vi "CrossedLine.vi"(0 "Xpoint1":dbl, 1 "Ypoint1":dbl, 4 "Xpoint2":dbl, 5 "Ypoint2":dbl, 6 "XpointC":dbl, 7 "YpointC":dbl, 8 "XpointP":dbl=-1.0, 9 "YpointP":dbl=-1.0) -> (12 "NextPriorX":dbl, 13 "NextPriorY":dbl, 17 "CrossedLine":bool)   [LabVIEW 2012]
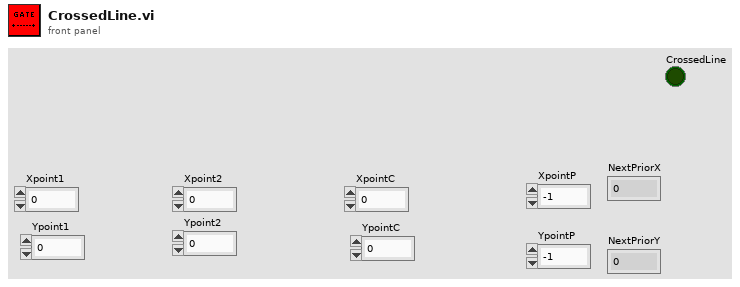
[diagram p1: front panel]
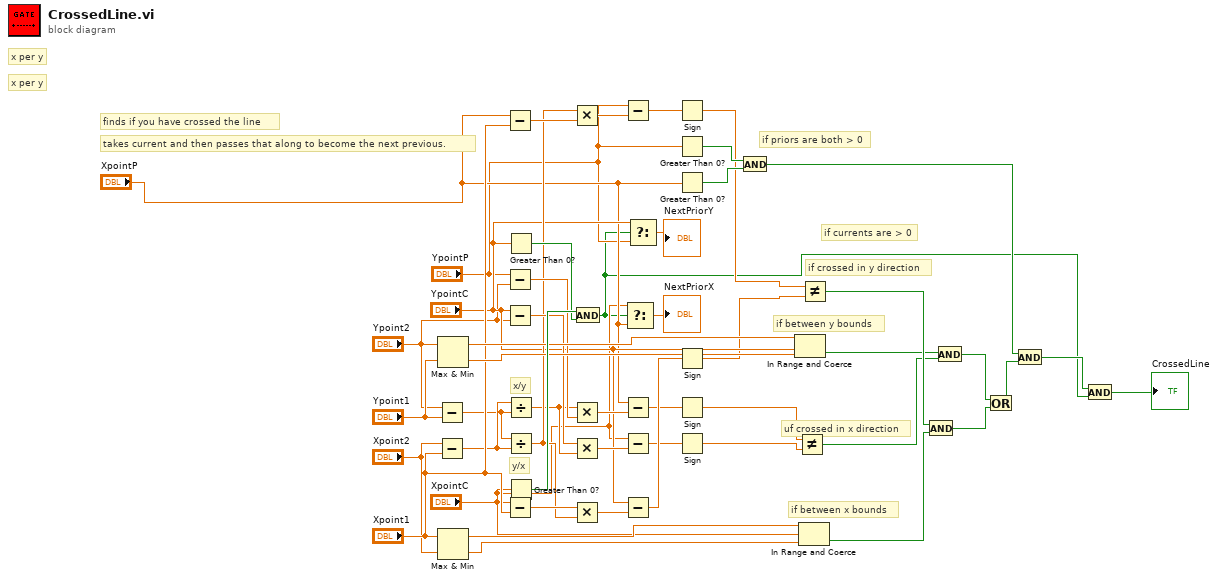
[diagram p0: block diagram]
diagram:
  # "if currents are > 0"
  # "uf crossed in x direction"
  # "if crossed in y direction"
  # "y/x"
  # "x/y"
  # "if between x bounds"
  # "if between y bounds"
  # "if priors are both > 0"
  # "x per y"
  # "finds if you have crossed the line"
  # "takes current and then passes that along to become the next previous."
  # "x per y"
  n1 = Subtract(x="Ypoint2", y="Ypoint1") -> (x-y=w21:dbl)
  n2 = Subtract(x="Xpoint2", y="Xpoint1") -> (x-y=w22:dbl)
  n3 = Max & Min(x="Ypoint2", y="Ypoint1") -> (max(x,y)=w37:dbl, min(x,y)=w36:dbl)
  n4 = Max & Min(x="Xpoint1", y="Xpoint2") -> (max(x,y)=w28:dbl, min(x,y)=w12:dbl)
  n5 = Subtract(x="XpointP", y="Xpoint1") -> (x-y=w48:dbl)
  n6 = Subtract(x="YpointP", y="Ypoint2") -> (x-y=w33:dbl)
  n7 = Subtract(x="YpointC", y="Ypoint2") -> (x-y=w34:dbl)
  n8 = Subtract(x="XpointC", y="Xpoint1") -> (x-y=w49:dbl)
  n9 = Greater Than 0?(x="YpointC") -> (x > 0?=w38:bool)
  n10 = Divide(x=w22, y=w21) -> (x/y=w20:dbl)
  n11 = Divide(x=w21, y=w22) -> (x/y=w25:dbl)
  n12 = Greater Than 0?(x="XpointC") -> (x > 0?=w39:bool)
  n13 = Multiply(x=w25, y=w48) -> (x*y=w46:dbl)
  n14 = Multiply(x=w20, y=w33) -> (x*y=w31:dbl)
  n15 = Multiply(x=w34, y=w20) -> (x*y=w32:dbl)
  n16 = Multiply(x=w49, y=w25) -> (x*y=w47:dbl)
  n17 = And(x=w39, y=w38) -> (x .and. y?=w2:bool)
  n18 = Subtract(x="YpointP", y=w46) -> (x-y=w44:dbl)
  n19 = Subtract(x="XpointP", y=w31) -> (x-y=w29:dbl)
  n20 = Subtract(x="XpointC", y=w32) -> (x-y=w30:dbl)
  n21 = Subtract(x="YpointC", y=w47) -> (x-y=w45:dbl)
  n22 = Select(t="XpointC", s=w2, f="XpointP") -> (s? t:f=→"NextPriorX":dbl)
  n23 = Select(t="YpointC", s=w2, f="YpointP") -> (s? t:f=→"NextPriorY":dbl)
  n24 = Sign(1:w44) -> (0:w16:dbl)
  n25 = Greater Than 0?(x="YpointP") -> (x > 0?=w40:bool)
  n26 = Greater Than 0?(x="XpointP") -> (x > 0?=w41:bool)
  n27 = Sign(1:w45) -> (0:w15:dbl)
  n28 = Sign(1:w29) -> (0:w13:dbl)
  n29 = Sign(1:w30) -> (0:w14:dbl)
  n30 = And(x=w40, y=w41) -> (x .and. y?=w4:bool)
  n31 = In Range and Coerce(upper limit=w37, x="YpointC", lower limit=w36) -> (In Range?=w8:bool)  [unwired: 1 out]
  n32 = Not Equal?(x=w13, y=w14) -> (x != y?=w9:bool)
  n33 = In Range and Coerce(upper limit=w28, x="XpointC", lower limit=w12) -> (In Range?=w10:bool)  [unwired: 1 out]
  n34 = Not Equal?(x=w16, y=w15) -> (x != y?=w11:bool)
  n35 = And(x=w11, y=w10) -> (x .and. y?=w7:bool)
  n36 = And(x=w8, y=w9) -> (x .and. y?=w6:bool)
  n37 = Or(x=w6, y=w7) -> (x .or. y?=w5:bool)
  n38 = And(x=w4, y=w5) -> (x .and. y?=w3:bool)
  n39 = And(x=w3, y=w2) -> (x .and. y?=→"CrossedLine":bool)
